vi "外观 1.vi"(0 "Data In":T4 caption="数据输入", 2 "Display State In":T2 caption="显示状态输入", 3 "Container State":T3 caption="容器状态") -> (6 "Data Out":T4 caption="数据输出", 7 "Display State Out":T2 caption="显示状态输出", 8 "Action":T1 caption="动作")   [LabVIEW 2014, in "波形图_显示点坐标.xctl"]
uses:
  <vilib>/_xctls/Container State.ctl
  <vilib>/_xctls/Action.ctl
  <vilib>/_xctls/XControlSupport.lvlib
panel:
  out "坐标字符串":string
  out "波形图":dbl[][](graph)
  # "1. 放置组成XControl外观\n的控件。\n\n2. 根据控件调整窗口大小。\n\n3. 如XControl为固定大小，\n通过“VI属性->窗口外观”将窗口设置为无法调整大小。\n\n4.如需根据XControl自动调整控件大小，在“文件->VI属性->窗口大小”页面中勾选“调整窗口大小时缩放前面板上所有对象”复选框。 \n\n5. 显示程序框图并处理前面板上的控件事件。"
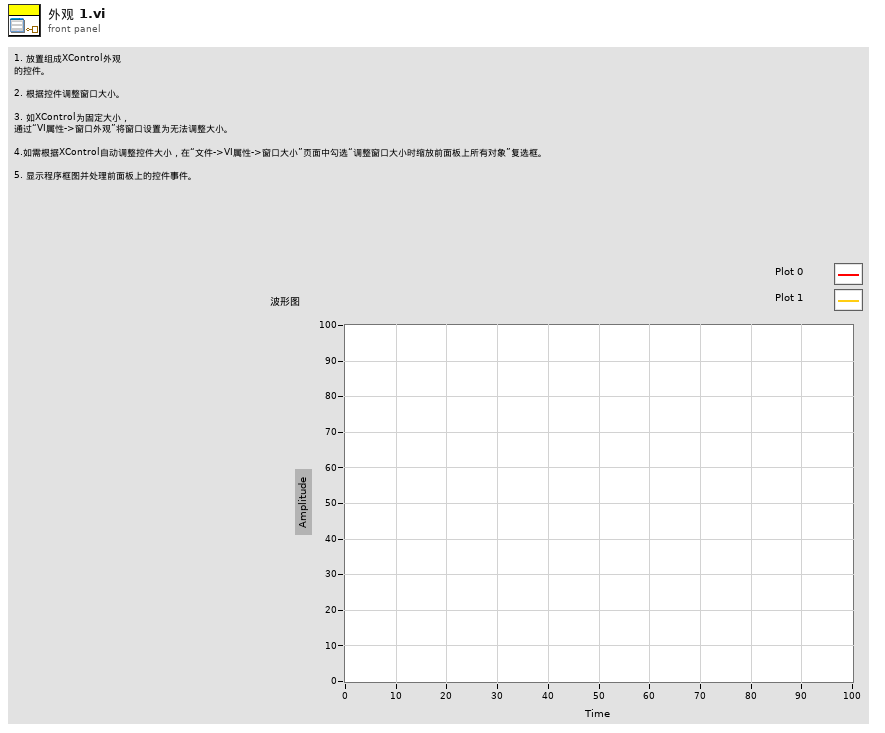
[diagram p1: front panel]
types:
  T1 = typedef "XControlSupport.lvlib/Action.ctl" = cluster{"Data Changed?":bool, "State Changed?":bool, "Action Name":string}
  T2 = typedef "波形图_显示点坐标.xctl/状态 1.ctl" = cluster{" 波形图":dbl[][]}
  T3 = typedef "XControlSupport.lvlib/Container State.ctl" = cluster{"Indicator?":bool, "Run Mode?":bool, " Refnum":refnum<vi>}
  T4 = typedef "波形图_显示点坐标.xctl/数据 1.ctl" = dbl[][]
  T5 = typedef "LVPoint32TypeDef.ctl" = cluster{"Horizontal":i32, "Vertical":i32}
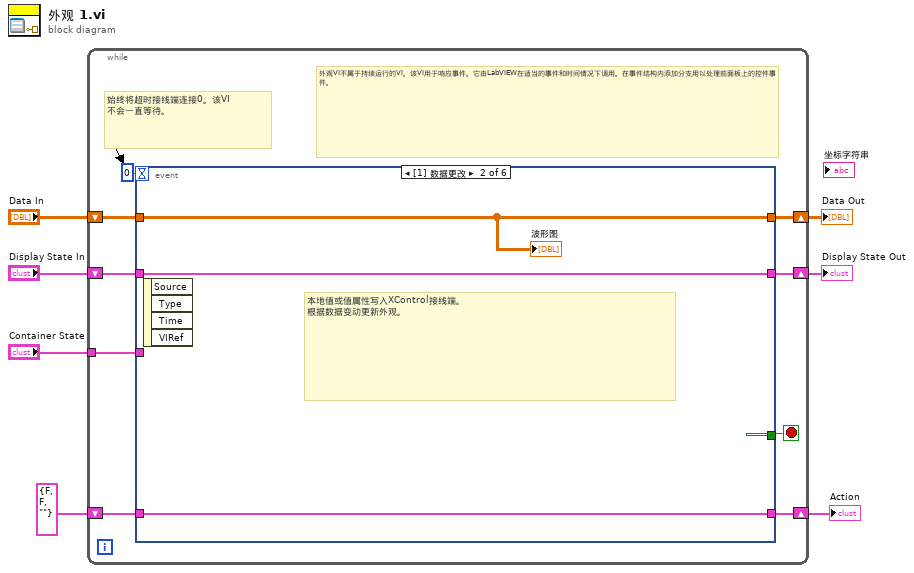
[diagram p0: block diagram]
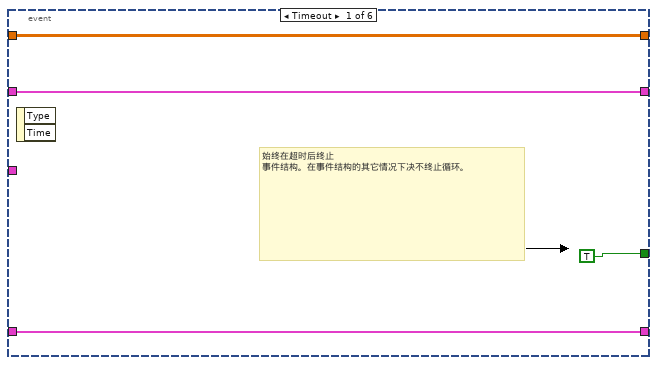
[diagram p2: hidden frame]
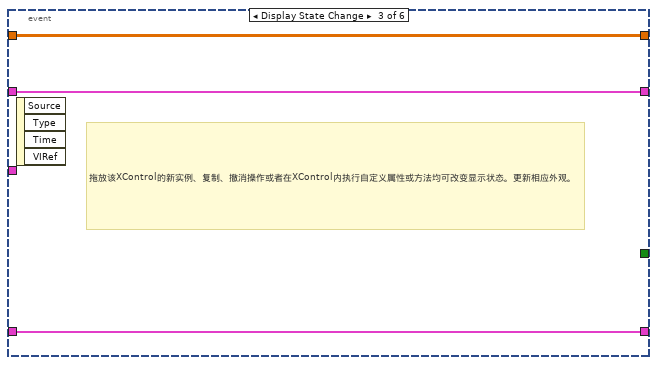
[diagram p3: hidden frame]
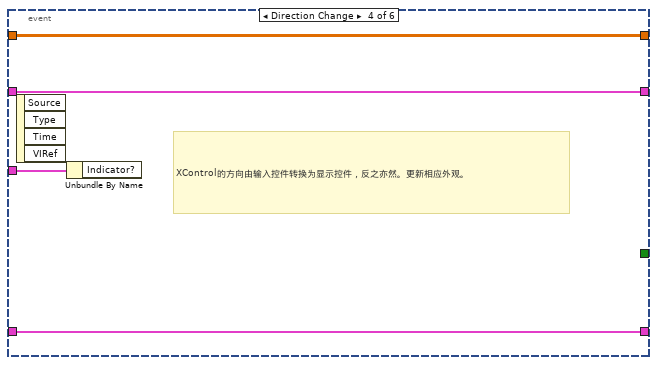
[diagram p4: hidden frame]
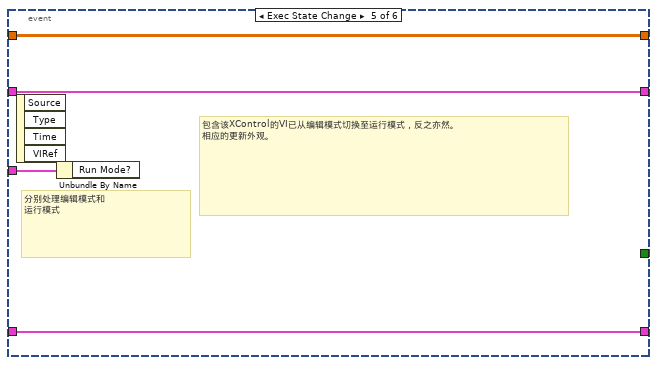
[diagram p5: hidden frame]
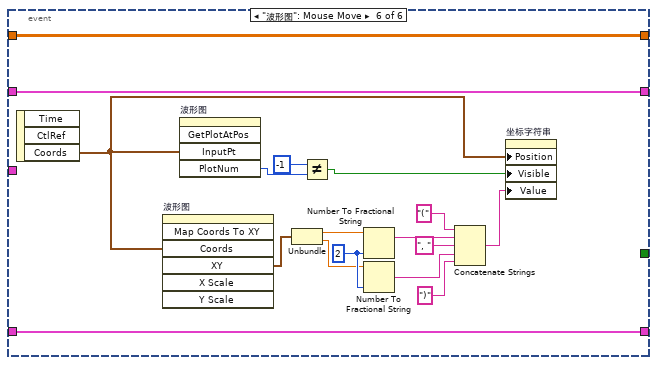
[diagram p6: hidden frame]
diagram:
  n1 = while {
    shift-right: [w15] -> w4
    shift-left: "Display State In" -> [w16]
    tunnel: "Container State" -> [w12]
    shift-right: [w10] -> w7
    shift-left: "Data In" -> [w11]
    shift-right: [w8] -> w2
    shift-left: T1 {"Data Changed?"=FALSE, "State Changed?"=FALSE, "Action Name"=""} ("Action") -> [w9]
    stop <- w14 stop-if-true
    # "外观VI不属于持续运行的VI。该VI用于响应事件。它由LabVIEW在适当的事件和时间情况下调用。在事件结构内添加分支用以处理前面板上的控件事件。"
    # "始终将超时接线端连接0。该VI\n不会一直等待。"
    n2 = event shown="[1] 数据更改" {
      selector: _ -> [_ _ _ _ _ _]
      dyn-events: _ -> [_ _ _ _ _ _]
      timeout: 0 -> [_ _ _ _ _ _]
      tunnel: w16 -> [w18 w23 w26 w29 w33 w51]
      tunnel: [w18 w23 w26 w29 w33 w51] -> w15
      tunnel: [TRUE _ _ _ _ _] -> w14
      tunnel: w12 -> [_ _ _ w30 w34 _]
      tunnel: w11 -> [w17 w21 w25 w28 w32 w50]
      tunnel: [w17 w21 w25 w28 w32 w50] -> w10
      tunnel: [w19 w22 w24 w27 w31 w49] -> w8
      tunnel: w9 -> [w19 w22 w24 w27 w31 w49]
      event Timeout {
        # "始终在超时后终止\n事件结构。在事件结构的其它情况下决不终止循环。"
        n3 = event-data() -> ()  [unwired: 1 in, 2 out]
      }
      event Data Change {
        # "本地值或值属性写入XControl接线端。\n根据数据变动更新外观。"
        n4 = event-data() -> ()  [unwired: 1 in, 4 out]
        "波形图" <- w21
      }
      event Display State Change {
        # "拖放该XControl的新实例、复制、撤消操作或者在XControl内执行自定义属性或方法均可改变显示状态。更新相应外观。"
        n5 = event-data() -> ()  [unwired: 1 in, 4 out]
      }
      event Direction Change {
        # "XControl的方向由输入控件转换为显示控件，反之亦然。更新相应外观。"
        n6 = event-data() -> ()  [unwired: 1 in, 4 out]
        n7 = Unbundle By Name(w30) -> ()  [unwired: 1 out]
      }
      event Exec State Change {
        # "包含该XControl的VI已从编辑模式切换至运行模式，反之亦然。\n相应的更新外观。"
        # "分别处理编辑模式和\n运行模式"
        n8 = event-data() -> ()  [unwired: 1 in, 4 out]
        n9 = Unbundle By Name(w34) -> ()  [unwired: 1 out]
      }
      event "波形图": Mouse Move {
        w44 = i16 2 ("precision (6)")
        n10 = event-data() -> ("Coords"=w45:T5)  [unwired: 1 in, 2 out]
        n11 = invoke on="波形图" class="WFGraph (严格)" method="Map Coords To XY"("Coords"=w45) -> ("XY"=w36:cluster{"X":dbl, "Y":dbl})  [unwired: 6 in, 6 out]
        n12 = invoke on="波形图" class="WFGraph (严格)" method="GetPlotAtPos"("InputPt"=w45) -> ("PlotNum"=w48:i32)  [unwired: 4 in, 4 out]
        n13 = Unbundle(w36) -> ("X"=w37:dbl, "Y"=w38:dbl)
        n14 = Not Equal?(x=-1, y=w48) -> (x != y?=w46:bool)
        n15 = Number To Fractional String(number=w37, precision (6)=w44) -> (F-format string=w39:string)  [unwired: 2 in]
        n16 = Number To Fractional String(number=w38, precision (6)=w44) -> (F-format string=w42:string)  [unwired: 2 in]
        n17 = Concatenate Strings("(" ("字符串"), w39, ", ", w42, ")" ("字符串")) -> (w35:string)
        n18 = property on="坐标字符串" class="Str"("Position"=w45, "Visible"=w46, "Value"=w35) -> ()  [unwired: 2 in, 2 out]
      }
    }
  }
  "Display State Out" <- w4
  "Data Out" <- w7
  "Action" <- w2
